vi "FirmwareUpdater.vi"() -> ()   [LabVIEW 2012]
uses:
  Type/_Updater Tasks.ctl
  Type/_Log Command.ctl
  Type/_RT Command.ctl
  Type/_RT Configuration 2.ctl
  <vilib>/Utility/config.llb/Read Key (String).vi
  <vilib>/Utility/config.llb/Read Key (Boolean).vi
  Configuration/_Global Configuration.vi
  <vilib>/Utility/config.llb/NI_LVConfig.lvlib
panel:
  in  "Done":bool
  out "IP Address:":string
  out "Messages":string
  out "Current Task":string
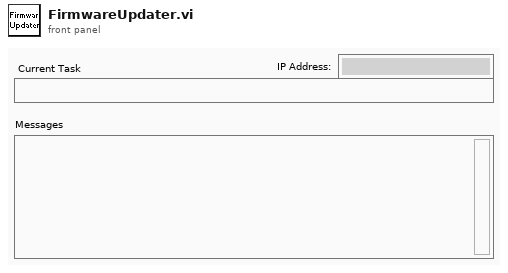
[diagram p1: front panel]
types:
  T1 = typedef "_Updater Tasks.ctl" = enum16{"Initialize", "ValidateFirmware", "MakeConnection", "UpdateFirmware", "LoadTable", "Error", "Done"}
  T2 = typedef "_Log Command.ctl" = enum16{"No Command", "Open", "Read", "Write", "Close", "Check Size"}
  T3 = typedef "_RT Command.ctl" = enum16{"Start", "Stop", "Runtime Update", "Get Data", "Get Info", "Get Status", "Get Param", "Get Config", "Get Table", "Read ADC", "Set Oscillator", "Update Config", "Update Table", "Set All Pol", "Set Pol and DC", "Set Max Mass", "Toggle RP", "Toggle EL", "Set PIC", "Initialize Turbo", "Send Turbo Comm", "Close Turbo", "P1", "P2", "P3", "Send Serial", "Set LC Out", "Get LC In", "Read VAC", "Test Table", "Toggle Power", "Get Startup", "Set Startup", "Get ADC Table", "Set ADC Table", "Get Brief Status", "Get Detail Status", "Auxiliary Update", "Set CC Logics", "Set CC Input Logics", "Ignore Error"}
  T4 = cluster{"UpdaterTasks":T1, "Error":string, "Messages":string, "Config":bool, "CalRes":bool, "ADC":bool}
  T5 = typedef "NI_LVConfig.lvlib/Config Data RefNum.ctl" = refnum<k1>
  T6 = cluster{"IP Address:":string, string, "appended path":path, "Source":enum32{"RT Target", "Folder"}}
  T7 = typedef "_RT Instrument 2.ctl" = cluster{"Table":T8[], "Instrument":string[]}
  T8 = typedef "_RT Configuration 2.ctl" = cluster{"Name":string, "Ch#":u8, "Min":dbl, "Max":dbl, "Def+":dbl, "Def-":dbl, "Offset":dbl, "Slope":dbl, "Type":u8, "Description":string, "SettleT":dbl}
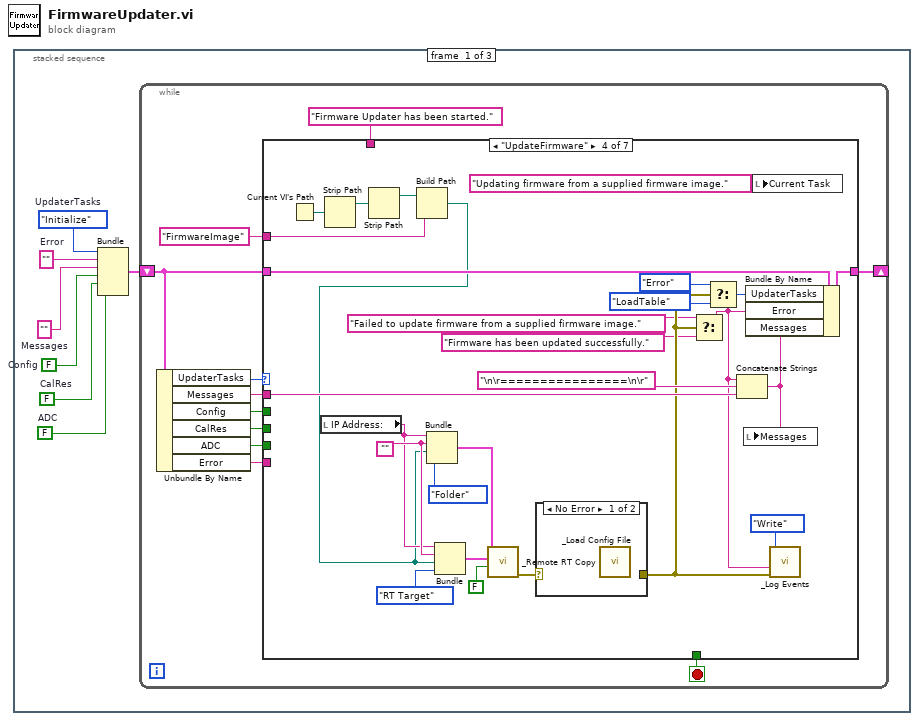
[diagram p0: block diagram]
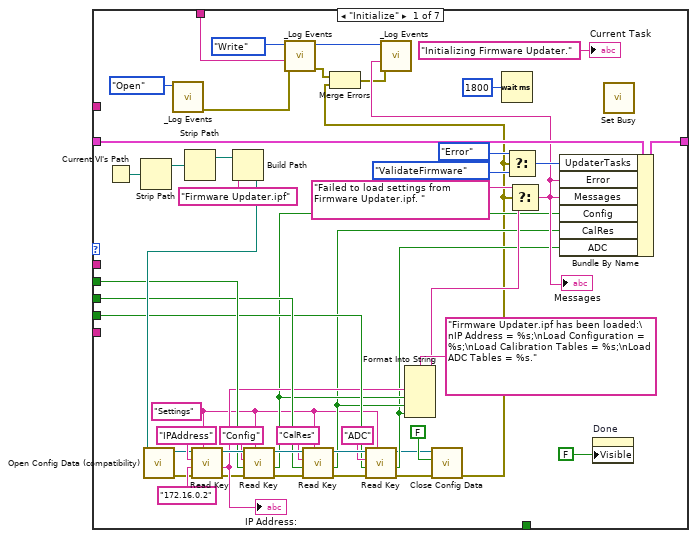
[diagram p2: hidden frame]
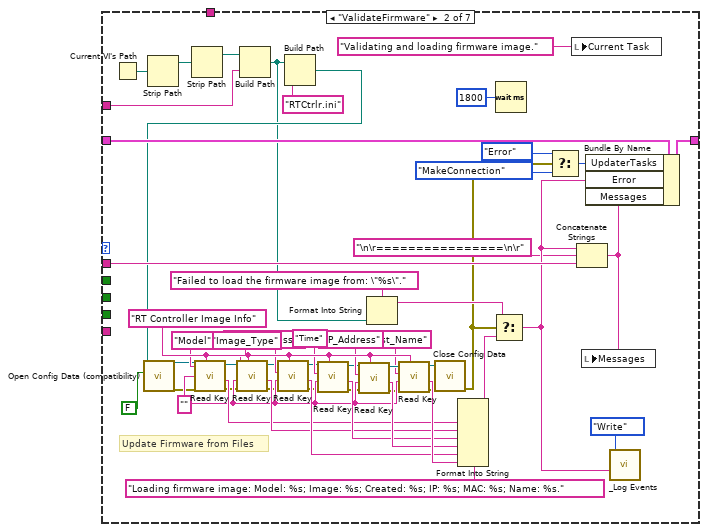
[diagram p3: hidden frame]
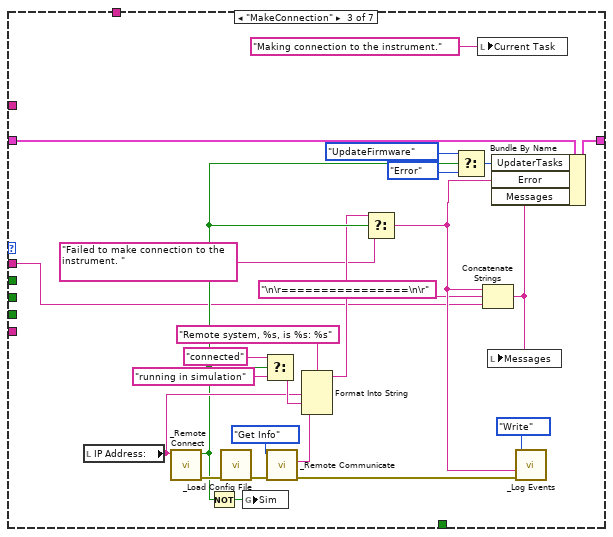
[diagram p4: hidden frame]
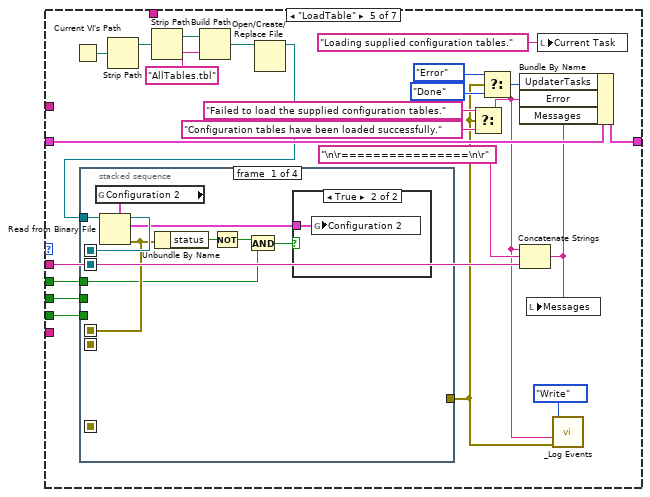
[diagram p6: hidden frame]
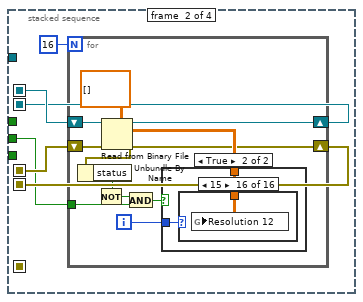
[diagram p8: hidden frame]
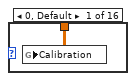
[diagram p10: hidden frame]
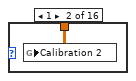
[diagram p11: hidden frame]
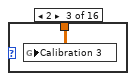
[diagram p12: hidden frame]
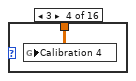
[diagram p13: hidden frame]
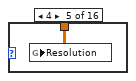
[diagram p14: hidden frame]
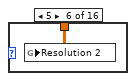
[diagram p15: hidden frame]
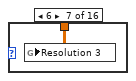
[diagram p16: hidden frame]
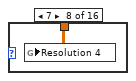
[diagram p17: hidden frame]
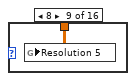
[diagram p18: hidden frame]
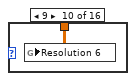
[diagram p19: hidden frame]
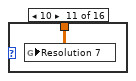
[diagram p20: hidden frame]
diagram:
  n1 = stacked-sequence {
    frame #0 {
      w1 = FALSE  # ADC
      w2 = FALSE  # CalRes
      w3 = FALSE  # Config
      w4 = ""  # Messages
      w7 = _Updater_Tasks."Initialize"  # UpdaterTasks
      w6 = ""  # Error
      n2 = Bundle("UpdaterTasks"=w7, "Error"=w6, "Messages"=w4, "Config"=w3, "CalRes"=w2, "ADC"=w1) -> (w5:T4)  [unwired: 1 out]
      n3 = while {
        shift-right: [w15] -> _
        shift-left: w5 -> [w16]
        stop <- w9 stop-if-true
        n4 = Unbundle By Name(w16) -> ("UpdaterTasks"=w18:T1, "Messages"=w14:string, "Config"=w13:bool, "CalRes"=w12:bool, "ADC"=w11:bool, "Error"=w10:string)
        n5 = case shown="\"UpdateFirmware\"" w18 {
          tunnel: "Firmware Updater has been started." ("string") -> [w64 _ _ _ _ _ _]
          tunnel: w16 -> [w63 w119 w144 w171 w195 w282 w287]
          tunnel: [w62 w118 w143 w170 w194 w281 w287] -> w15
          tunnel: w14 -> [_ w111 w121 w168 w192 _ _]
          tunnel: w13 -> [w40 _ _ _ w176 _ _]
          tunnel: w12 -> [w36 _ _ _ w175 _ _]
          tunnel: w11 -> [w35 _ _ _ w174 _ _]
          tunnel: w10 -> [_ _ _ _ _ w277 _]
          tunnel: [_ _ _ _ _ _ w286] -> w9
          tunnel: "FirmwareImage" -> [_ w67 _ w145 _ _ _]
          frame "Initialize" {
            w25 = "Settings" ("section")
            w46 = _Log_Command."Write" ("File Command")
            n6 = Current VI's Path() -> (path=w61:path)
            n7 = Strip Path(path=w61) -> (stripped path=w60:path)  [unwired: 1 out]
            n8 = call "_Log Events.vi"("Log Command"=_Log_Command."Open" ("File Command")) -> ("error out"=w66:errorcluster)  [unwired: 3 in, 4 out]
            n9 = Strip Path(path=w60) -> (stripped path=w59:path)  [unwired: 1 out]
            n10 = Build Path(base path=w59, name or relative path="Firmware Updater.ipf") -> (appended path=w58:path)
            n11 = call <vilib>:"Open Config Data (compatibility).vi"("configuration file path"=w58) -> ("error out"=w52:errorcluster, "refnum"=w53:T5)  [unwired: 8 in, 1 out]
            n12 = call-poly <vilib>:"Read Key.vi"("section"=w25, "error in (no error)"=w52, "default value"="172.16.0.2", "key"="IPAddress" ("section"), "refnum"=w53) -> ("error out"=w26:errorcluster, "value"=w34:string, "refnum out"=w43:T5)  [unwired: 1 in, 3 out]
            "IP Address:" <- w34
            n13 = call-poly <vilib>:"Read Key.vi"("section"=w25, "error in (no error)"=w26, "default value"=w40, "key"="Config" ("section"), "refnum"=w43) -> ("error out"=w23:errorcluster, "value"=w31:bool, "refnum out"=w42:T5)  [unwired: 4 out]
            n14 = call "_Log Events.vi"("error in (no error)"=w66, "Event"=w64, "Log Command"=w46) -> ("error out"=w28:errorcluster)  [unwired: 1 in, 4 out]
            n15 = call-poly <vilib>:"Read Key.vi"("section"=w25, "error in (no error)"=w23, "default value"=w36, "key"="CalRes" ("section"), "refnum"=w42) -> ("error out"=w22:errorcluster, "value"=w30:bool, "refnum out"=w41:T5)  [unwired: 4 out]
            n16 = call-poly <vilib>:"Read Key.vi"("section"=w25, "error in (no error)"=w22, "default value"=w35, "key"="ADC" ("section"), "refnum"=w41) -> ("error out"=w21:errorcluster, "value"=w29:bool, "refnum out"=w24:T5)  [unwired: 4 out]
            n17 = Format Into String(format string="Firmware Updater.ipf has been loaded:\nIP Address = %s;\nLoad Configuration = %s;\nLoad Calibration Tables = %s;\nLoad ADC Tables = %s.", w34, w31, w30, w29) -> (resulting string=w32:string)  [unwired: 2 in, 1 out]
            n18 = call <vilib>:"Close Config Data.vi"("error in (no error)"=w21, "write file if changed (T)"=FALSE ("write configuration file? (T)"), "refnum"=w24) -> ("error out"=w20:errorcluster)  [unwired: 8 out]
            n19 = Merge Errors(w28, w20) -> (w27:errorcluster)
            n20 = Wait (ms)(milliseconds to wait=u32 1800) -> ()  [unwired: 1 out]
            n21 = Select(t=_Updater_Tasks."Error" ("UpdaterTasks"), s=w20, f=_Updater_Tasks."ValidateFirmware" ("UpdaterTasks")) -> (s? t:f=w48:T1)
            n22 = Select(t="Failed to load settings from Firmware Updater.ipf. ", s=w20, f=w32) -> (s? t:f=w45:string)
            "Messages" <- w45
            n23 = call "_Log Events.vi"("error in (no error)"=w27, "Event"=w45, "Log Command"=w46) -> ()  [unwired: 1 in, 5 out]
            n24 = Bundle By Name(cluster=w63, "UpdaterTasks"=w48, "Error"=w45, "Messages"=w45, "Config"=w31, "CalRes"=w30, "ADC"=w29) -> (w62:T4)
            n25 = property on="Done" class="Bool"("Visible"=FALSE) -> ()  [unwired: 2 in, 2 out]
            n26 = call <vilib>:"Set Busy.vi"() -> ()  [unwired: 4 in, 8 out]
            "Current Task" <- "Initializing Firmware Updater." ("Current Task")
          }
          frame "ValidateFirmware" {
            w97 = ""
            w106 = "RT Controller Image Info" ("section")
            # "Update Firmware from Files"
            n27 = Current VI's Path() -> (path=w110:path)
            n28 = Strip Path(path=w110) -> (stripped path=w109:path)  [unwired: 1 out]
            n29 = Strip Path(path=w109) -> (stripped path=w108:path)  [unwired: 1 out]
            n30 = Build Path(base path=w108, name or relative path=w67) -> (appended path=w73:path)
            n31 = Build Path(base path=w73, name or relative path="RTCtrlr.ini") -> (appended path=w75:path)
            n32 = call <vilib>:"Open Config Data (compatibility).vi"("create file if necessary (T)"=FALSE ("create file if necessary? (T)"), "configuration file path"=w75) -> ("error out"=w77:errorcluster, "refnum"=w76:T5)  [unwired: 7 in, 1 out]
            n33 = call-poly <vilib>:"Read Key.vi"("section"=w106, "error in (no error)"=w77, "default value"=w97, "key"="Model", "refnum"=w76) -> ("error out"=w80:errorcluster, "value"=w99:string, "refnum out"=w79:T5)  [unwired: 1 in, 3 out]
            n34 = call-poly <vilib>:"Read Key.vi"("section"=w106, "error in (no error)"=w80, "default value"=w97, "key"="Image_Type", "refnum"=w79) -> ("error out"=w83:errorcluster, "value"=w100:string, "refnum out"=w82:T5)  [unwired: 1 in, 3 out]
            n35 = call-poly <vilib>:"Read Key.vi"("section"=w106, "error in (no error)"=w83, "default value"=w97, "key"="MAC_Address", "refnum"=w82) -> ("error out"=w87:errorcluster, "value"=w103:string, "refnum out"=w86:T5)  [unwired: 1 in, 3 out]
            n36 = call-poly <vilib>:"Read Key.vi"("section"=w106, "error in (no error)"=w87, "default value"=w97, "key"="Time", "refnum"=w86) -> ("error out"=w94:errorcluster, "value"=w101:string, "refnum out"=w93:T5)  [unwired: 1 in, 3 out]
            n37 = call-poly <vilib>:"Read Key.vi"("section"=w106, "error in (no error)"=w94, "default value"=w97, "key"="IP_Address", "refnum"=w93) -> ("error out"=w96:errorcluster, "value"=w102:string, "refnum out"=w95:T5)  [unwired: 1 in, 3 out]
            n38 = Format Into String(format string="Failed to load the firmware image from: \"%s\"." ("t"), w73) -> (resulting string=w72:string)  [unwired: 2 in, 1 out]
            n39 = call-poly <vilib>:"Read Key.vi"("section"=w106, "error in (no error)"=w96, "default value"=w97, "key"="Host_Name", "refnum"=w95) -> ("error out"=w89:errorcluster, "value"=w104:string, "refnum out"=w88:T5)  [unwired: 1 in, 3 out]
            n40 = call <vilib>:"Close Config Data.vi"("error in (no error)"=w89, "refnum"=w88) -> ("error out"=w71:errorcluster)  [unwired: 1 in, 8 out]
            n41 = Format Into String(format string="Loading firmware image: Model: %s; Image: %s; Created: %s; IP: %s; MAC: %s; Name: %s.", w99, w100, w101, w102, w103, w104) -> (resulting string=w92:string)  [unwired: 2 in, 1 out]
            n42 = Select(t=w72, s=w71, f=w92) -> (s? t:f=w70:string)
            n43 = Wait (ms)(milliseconds to wait=u32 1800) -> ()  [unwired: 1 out]
            n44 = Select(t=_Updater_Tasks."Error" ("UpdaterTasks"), s=w71, f=_Updater_Tasks."MakeConnection" ("UpdaterTasks")) -> (s? t:f=w115:T1)
            n45 = local write "Current Task"("Validating and loading firmware image." ("Current Task")) -> ()
            n46 = Concatenate Strings(w70, "\n\r================\n\r" ("string"), w111) -> (w112:string)
            n47 = local write "Messages"(w112) -> ()
            n48 = Bundle By Name(cluster=w119, "UpdaterTasks"=w115, "Error"=w70, "Messages"=w112) -> (w118:T4)
            n49 = call "_Log Events.vi"("Event"=w70, "Log Command"=_Log_Command."Write" ("File Command")) -> ()  [unwired: 2 in, 5 out]
          }
          frame "MakeConnection" {
            n50 = local read "IP Address:"() -> (w130:string)
            n51 = call "_Remote Connect.vi"("IP Address"=w130) -> ("error out"=w139:errorcluster, "TCP"=w126:bool)  [unwired: 1 in, 4 out]
            n52 = Not(x=w126) -> (.not. x?=w131:bool)
            n53 = call "_Load Config File.vi"("error in (no error)"=w139) -> ("error out"=w141:errorcluster)  [unwired: 6 out]
            n54 = global write "_Global Configuration.vi" "Sim"(w131) -> ()
            n55 = Select(t="connected", s=w126, f="running in simulation") -> (s? t:f=w133:string)
            n56 = call "_Remote Communicate.vi"("error in (no error)"=w141, "Command"=_RT_Command."Get Info") -> ("error out"=w140:errorcluster, "Info"=w138:string)  [unwired: 4 in, 2 out]
            n57 = Format Into String(format string="Remote system, %s, is %s: %s", w130, w133, w138) -> (resulting string=w125:string)  [unwired: 2 in, 1 out]
            n58 = Select(t=w125, s=w126, f="Failed to make connection to the instrument. ") -> (s? t:f=w122:string)
            n59 = Select(t=_Updater_Tasks."UpdateFirmware" ("UpdaterTasks"), s=w126, f=_Updater_Tasks."Error" ("UpdaterTasks")) -> (s? t:f=w129:T1)
            n60 = local write "Current Task"("Making connection to the instrument." ("Current Task")) -> ()
            n61 = Concatenate Strings(w122, "\n\r================\n\r" ("string"), w121) -> (w124:string)
            n62 = local write "Messages"(w124) -> ()
            n63 = Bundle By Name(cluster=w144, "UpdaterTasks"=w129, "Error"=w122, "Messages"=w124) -> (w143:T4)
            n64 = call "_Log Events.vi"("error in (no error)"=w140, "Event"=w122, "Log Command"=_Log_Command."Write" ("File Command")) -> ()  [unwired: 1 in, 5 out]
          }
          frame "UpdateFirmware" {
            w165 = ""
            n65 = Current VI's Path() -> (path=w157:path)
            n66 = local read "IP Address:"() -> (w158:string)
            n67 = Strip Path(path=w157) -> (stripped path=w156:path)  [unwired: 1 out]
            n68 = Strip Path(path=w156) -> (stripped path=w155:path)  [unwired: 1 out]
            n69 = Build Path(base path=w155, name or relative path=w145) -> (appended path=w154:path)
            n70 = Bundle("IP Address:"=w158, w165, "appended path"=w154, "Source"=enum32{"RT Target", "Folder"}."Folder") -> (w161:T6)  [unwired: 1 out]
            n71 = Bundle("IP Address:"=w158, w165, "appended path"=w154, "Source"=enum32{"RT Target", "Folder"}."RT Target") -> (w160:T6)  [unwired: 1 out]
            n72 = call "_Remote RT Copy.vi"("Copy software only"=FALSE, "Image Destination"=w160, "Image Source"=w161) -> ("Error Out"=w159:errorcluster)  [unwired: 1 in, 5 out]
            n73 = case shown="No Error" w159 {
              selector: w159 -> [_ w172]
              tunnel: [_ w172] -> w149
              frame No Error {
                n74 = call "_Load Config File.vi"() -> ()  [unwired: 1 in, 7 out]
              }
              frame Error {
              }
            }
            n75 = Select(t="Failed to update firmware from a supplied firmware image.", s=w149, f="Firmware has been updated successfully.") -> (s? t:f=w146:string)
            n76 = Select(t=_Updater_Tasks."Error" ("UpdaterTasks"), s=w149, f=_Updater_Tasks."LoadTable" ("UpdaterTasks")) -> (s? t:f=w151:T1)
            n77 = Concatenate Strings(w146, "\n\r================\n\r" ("string"), w168) -> (w150:string)
            n78 = local write "Messages"(w150) -> ()
            n79 = Bundle By Name(cluster=w171, "UpdaterTasks"=w151, "Error"=w146, "Messages"=w150) -> (w170:T4)
            n80 = local write "Current Task"("Updating firmware from a supplied firmware image.") -> ()
            n81 = call "_Log Events.vi"("error in (no error)"=w149, "Event"=w146, "Log Command"=_Log_Command."Write" ("File Command")) -> ()  [unwired: 1 in, 5 out]
          }
          frame "LoadTable" {
            n82 = Current VI's Path() -> (path=w189:path)
            n83 = Strip Path(path=w189) -> (stripped path=w188:path)  [unwired: 1 out]
            n84 = Strip Path(path=w188) -> (stripped path=w187:path)  [unwired: 1 out]
            n85 = Build Path(base path=w187, name or relative path="AllTables.tbl") -> (appended path=w178:path)
            n86 = Open/Create/Replace File(file path (use dialog)=w178) -> (refnum out=w177:refnum<file>)  [unwired: 5 in, 2 out]
            n87 = stacked-sequence {
              seq-local: [w202 _ _ _] -> [_ w210 _ _]
              seq-local: [_ w208 _ _] -> [_ _ w251 _]
              seq-local: [w201 _ _ _] -> [_ w211 _ _]
              seq-local: [_ w207 _ _] -> [_ _ w250 _]
              seq-local: [_ _ w241 _] -> [_ _ _ w263]
              tunnel: w177 -> [w204 _ _ _]
              tunnel: w176 -> [w198 _ _ w260]
              tunnel: w175 -> [_ w206 _ w259]
              tunnel: w174 -> [_ _ w245 _]
              tunnel: [_ _ _ w261] -> w173
              frame #0 {
                n88 = global read "_Global Configuration.vi" "Configuration 2"() -> (w203:T7)
                n89 = Read from Binary File(5:w203, 11:w204) -> (0:w201:errorcluster, 2:w196:T7, 3:w202:refnum<file>)  [unwired: 1 in, 4 out]
                n90 = Unbundle By Name(w201) -> ("status"=w200:bool)
                n91 = Not(x=w200) -> (.not. x?=w199:bool)
                n92 = And(x=w199, y=w198) -> (x .and. y?=w197:bool)
                n93 = case shown="True" w197 {
                  tunnel: w196 -> [_ w205]
                  frame False {
                  }
                  frame True {
                    n94 = global write "_Global Configuration.vi" "Configuration 2"(w205) -> ()
                  }
                }
              }
              frame #1 {
                n95 = for {
                  N: 16 -> [_]
                  shift-right: [w218] -> w208
                  shift-left: w210 -> [w222]
                  shift-right: [w216] -> w207
                  shift-left: w211 -> [w221]
                  tunnel: w206 -> [w213]
                  i -> [w217]
                  n96 = Read from Binary File(5:dbl[][] [] ("Cal-"), 8:w221, 11:w222) -> (0:w216:errorcluster, 2:w219:dbl[][], 3:w218:refnum<file>)  [unwired: 4 out]
                  n97 = Unbundle By Name(w216) -> ("status"=w215:bool)
                  n98 = Not(x=w215) -> (.not. x?=w214:bool)
                  n99 = And(x=w214, y=w213) -> (x .and. y?=w212:bool)
                  n100 = case shown="True" w212 {
                    tunnel: w219 -> [_ w223]
                    tunnel: w217 -> [_ w224]
                    frame False {
                    }
                    frame True {
                      n101 = case shown="15" w224 {
                        tunnel: w223 -> [w225 w226 w227 w228 w229 w230 w231 w232 w233 w234 w235 w236 w237 w238 w239 w240]
                        frame 0, Default {
                          n102 = global write "_Global Configuration.vi" "Calibration"(w225) -> ()
                        }
                        frame 1 {
                          n103 = global write "_Global Configuration.vi" "Calibration 2"(w226) -> ()
                        }
                        frame 2 {
                          n104 = global write "_Global Configuration.vi" "Calibration 3"(w227) -> ()
                        }
                        frame 3 {
                          n105 = global write "_Global Configuration.vi" "Calibration 4"(w228) -> ()
                        }
                        frame 4 {
                          n106 = global write "_Global Configuration.vi" "Resolution"(w229) -> ()
                        }
                        frame 5 {
                          n107 = global write "_Global Configuration.vi" "Resolution 2"(w230) -> ()
                        }
                        frame 6 {
                          n108 = global write "_Global Configuration.vi" "Resolution 3"(w231) -> ()
                        }
                        frame 7 {
                          n109 = global write "_Global Configuration.vi" "Resolution 4"(w232) -> ()
                        }
                        frame 8 {
                          n110 = global write "_Global Configuration.vi" "Resolution 5"(w233) -> ()
                        }
                        frame 9 {
                          n111 = global write "_Global Configuration.vi" "Resolution 6"(w234) -> ()
                        }
                        frame 10 {
                          n112 = global write "_Global Configuration.vi" "Resolution 7"(w235) -> ()
                        }
                        frame 11 {
                          n113 = global write "_Global Configuration.vi" "Resolution 8"(w236) -> ()
                        }
                        frame 12 {
                          n114 = global write "_Global Configuration.vi" "Resolution 9"(w237) -> ()
                        }
                        frame 13 {
                          n115 = global write "_Global Configuration.vi" "Resolution 10"(w238) -> ()
                        }
                        frame 14 {
                          n116 = global write "_Global Configuration.vi" "Resolution 11"(w239) -> ()
                        }
                        frame 15 {
                          n117 = global write "_Global Configuration.vi" "Resolution 12"(w240) -> ()
                        }
                      }
                    }
                  }
                }
              }
              frame #2 {
                w252 = T8[] []  # ADC Table
                n118 = Read from Binary File(5:w252, 8:w250, 11:w251) -> (0:w242:errorcluster, 2:w243:T8[])  [unwired: 5 out]
                n119 = Unbundle By Name(w242) -> ("status"=w248:bool)
                n120 = Array Size(array=w243) -> (size(s)=w249:i32)
                n121 = Greater Than 0?(x=w249) -> (x > 0?=w247:bool)
                n122 = Not(x=w248) -> (.not. x?=w246:bool)
                n123 = Compound Arithmetic op=AND(w247, w246, w245) -> (w244:bool)
                n124 = case shown="True" w244 {
                  tunnel: w243 -> [_ w258]
                  tunnel: [w253 w255] -> w241
                  tunnel: w242 -> [w253 w254]
                  frame False {
                  }
                  frame True {
                    n125 = Flatten To String(anything=w258) -> (data string=w256:string)  [unwired: 1 in, 4 out]
                    n126 = call "_Remote Communicate.vi"("String"=w256, "error in (no error)"=w254, "Command"=_RT_Command."Set ADC Table") -> ("error out"=w255:errorcluster)  [unwired: 3 in, 3 out]
                  }
                }
              }
              frame #3 {
                n127 = case shown="True" w260 {
                  tunnel: w263 -> [w272 w274]
                  tunnel: [w272 w273] -> w262
                  frame False {
                  }
                  frame True {
                    n128 = call "_Remote Communicate.vi"("error in (no error)"=w274, "Command"=_RT_Command."Update Config") -> ("error out"=w273:errorcluster)  [unwired: 4 in, 3 out]
                  }
                }
                n129 = case shown="True" w259 {
                  tunnel: w262 -> [w264 w267]
                  tunnel: [w264 w265] -> w261
                  frame False {
                  }
                  frame True {
                    n130 = for {
                      N: 16 -> [_]
                      shift-right: [w270] -> w265
                      shift-left: w267 -> [w268]
                      i -> [w269]
                      n131 = call "_Remote Communicate.vi"("error in (no error)"=w268, "DC Param"=w269, "Command"=_RT_Command."Update Table") -> ("error out"=w270:errorcluster)  [unwired: 3 in, 3 out]
                    }
                  }
                }
              }
            }
            n132 = Select(t="Failed to load the supplied configuration tables.", s=w173, f="Configuration tables have been loaded successfully.") -> (s? t:f=w179:string)
            n133 = Select(t=_Updater_Tasks."Error" ("UpdaterTasks"), s=w173, f=_Updater_Tasks."Done" ("UpdaterTasks")) -> (s? t:f=w183:T1)
            n134 = Concatenate Strings(w179, "\n\r================\n\r" ("string"), w192) -> (w182:string)
            n135 = Bundle By Name(cluster=w195, "UpdaterTasks"=w183, "Error"=w179, "Messages"=w182) -> (w194:T4)
            n136 = local write "Messages"(w182) -> ()
            n137 = local write "Current Task"("Loading supplied configuration tables.") -> ()
            n138 = call "_Log Events.vi"("error in (no error)"=w173, "Event"=w179, "Log Command"=_Log_Command."Write" ("File Command")) -> ()  [unwired: 1 in, 5 out]
          }
          frame "Error" {
            n139 = One Button Dialog(message=w277) -> ()  [unwired: 2 out]
            n140 = local write "Current Task"("Displaying error message." ("Current Task")) -> ()
            n141 = Bundle By Name(cluster=w282, "UpdaterTasks"=_Updater_Tasks."Done") -> (w281:T4)
            n142 = call "_Log Events.vi"("Event"="Error message displayed.", "Log Command"=_Log_Command."Write" ("File Command")) -> ()  [unwired: 2 in, 5 out]
          }
          frame "Done", Default {
            n143 = call <vilib>:"Unset Busy.vi"() -> ()  [unwired: 2 in, 10 out]
            n144 = while {
              tunnel: [w289] -> w286
              stop <- w289 stop-if-true
              n145 = event shown="[0] \"Done\": Value Change" {
                selector: _ -> [_ _]
                dyn-events: _ -> [_ _]
                timeout: _ -> [_ _]
                tunnel: ["Done" w291] -> w289
                event "Done": Value Change {
                  n146 = event-data() -> ()  [unwired: 6 out]
                }
                event Panel Close? {
                  w291 = TRUE ("Discard?")
                  n147 = event-data() -> ()  [unwired: 5 out]
                  n148 = event-data("Discard?"=w291) -> ()  [unwired: 1 in, 1 out]
                }
              }
            }
            n149 = call "_Log Events.vi"("Event"="Done-state reached.", "Log Command"=_Log_Command."Write" ("File Command")) -> ()  [unwired: 2 in, 5 out]
            n150 = property on="Done" class="Bool"("Visible"=TRUE) -> ()  [unwired: 2 in, 2 out]
            n151 = local write "Current Task"("Press the Done button to exit." ("Current Task")) -> ()
          }
        }
      }
    }
    frame #1 {
      n152 = call "_Log Events.vi"("Log Command"=_Log_Command."Close" ("File Command")) -> ()  [unwired: 3 in, 5 out]
    }
    frame #2 {
      w293 = TRUE  # release?
      n153 = Quit LabVIEW(quit? (T)=w293) -> ()
    }
  }
